vi "Initialize.vi"(8 "error in (no error)":errorcluster, 9 "Requestor":string, 10 "Requestee":string, 11 "Red Pitaya in":refnum<class "Red Pitaya.lvclass">) -> (0 "error out":errorcluster, 3 "Red Pitaya out":refnum<class "Red Pitaya.lvclass">)   [LabVIEW 2015, in "Red Pitaya.lvclass"]
uses:
  Red Pitaya.lvclass
  RP Command.ctl
  Mag Lab Measure/Hardware/Spectrum Analyzer/Spectrum Analyzer.lvclass/Spectrum Analyzer.ctl
  Red Pitaya.lvclass/Red Pitaya.ctl
  Mag Lab Measure/Hardware/Spectrum Analyzer/Read Frequencies.vi
  Mag Lab Measure/Hardware/Spectrum Analyzer/Read Duration.vi
  Mag Lab Measure/Hardware/Spectrum Analyzer/Spectrum Analyzer.lvclass
  Mag Lab Measure/Mag Lab Error Handler/Mag Lab Error Handler.lvclass
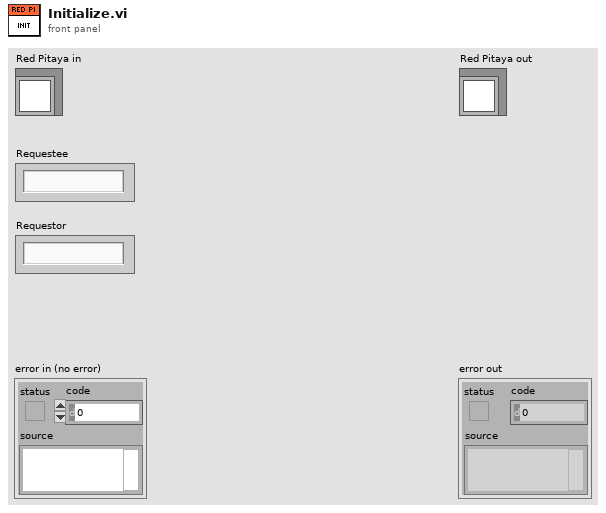
[diagram p1: front panel]
types:
  T1 = typedef "RP Command.ctl" = enum16{"Set frequency", "Arm and get data", "Stop server", "Get status", "Get temperature", "Set decimation", "Arm", "Software trigger", "Get whole buffer", "Get chunk", "System call", "Get config", "Set config", "Read FIFO", "Play pattern", "Set frequency batch"}
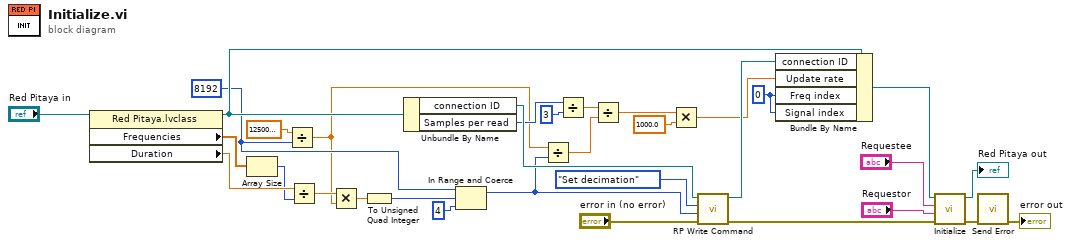
[diagram p0: block diagram]
diagram:
  w6 = 0 ("Freq index")
  w21 = u64 8192 ("x")
  n1 = property class="Red Pitaya.lvclass"(reference="Red Pitaya in") -> (reference out=w23:refnum<class "Red Pitaya.lvclass">, "Frequencies"=w28:dbl[], "Duration"=w5:dbl)  [unwired: 1 in, 1 out]
  n2 = Array Size(array=w28) -> (size(s)=w4:i32)
  n3 = Divide(x=125000000.0 ("y"), y=w21) -> (x/y=w11:dbl)
  n4 = Divide(x=w5, y=w4) -> (x/y=w26:dbl)
  n5 = Multiply(x=w26, y=w11) -> (x*y=w25:dbl)
  n6 = To Unsigned Quad Integer(1:w25) -> (0:w10:u64)
  n7 = Unbundle By Name(w23) -> ("connection ID"=w22:refnum<k5>, "Samples per read"=w13:i32)
  n8 = In Range and Coerce(upper limit=w21, x=w10, lower limit=u64 4 ("Command payload")) -> (coerced(x)=w3:u64)  [unwired: 1 out]
  n9 = Divide(x=w11, y=w3) -> (x/y=w8:dbl)
  n10 = Divide(x=w13, y=3) -> (x/y=w9:dbl)
  n11 = Divide(x=w9, y=w8) -> (x/y=w7:dbl)
  n12 = Multiply(x=w7, y=1000.0) -> (x*y=w2:dbl)
  n13 = call "RP Write Command.vi"("Error In"="error in (no error)", "Command payload"=w3, "Command number"=RP_Command."Set decimation", "connection ID"=w22) -> ("Error Out"=w18:errorcluster, "connection ID out"=w14:refnum<k5>)  [unwired: 5 in, 1 out]
  n14 = Bundle By Name(cluster=w23, "connection ID"=w14, "Update rate"=w2, "Freq index"=w6, "Signal index"=w6) -> (w15:refnum<class "Red Pitaya.lvclass">)
  n15 = call-parent "Initialize.vi"("error in (no error)"=w18, "Requestor"="Requestor", "Requestee"="Requestee", "Mag Lab Root in"=w15) -> ("error out"=w17:errorcluster, "Mag Lab Root out"=→"Red Pitaya out":refnum<class "Red Pitaya.lvclass">)  [unwired: 6 in]
  n16 = call "Send Error.vi"("error in (no error)"=w17) -> ("error out"=→"error out":errorcluster)  [unwired: 9 in, 1 out]
